vi "ByLuck.vi"(11 "InOrder":string[](array[string])) -> (3 "ByLuck":string)   [LabVIEW 2014]
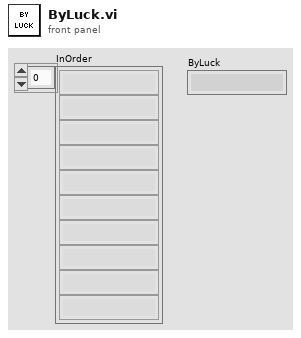
[diagram p1: front panel]
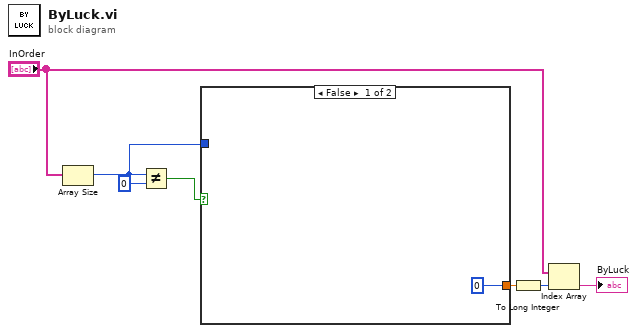
[diagram p0: block diagram]
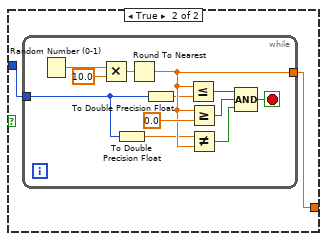
[diagram p2: hidden frame]
diagram:
  n1 = Array Size(array="InOrder") -> (size(s)=w3:i32)
  n2 = Not Equal?(x=w3, y=0) -> (x != y?=w4:bool)
  n3 = case shown="False" w4 {
    tunnel: [0 w10] -> w7
    tunnel: w3 -> [_ w9]
    frame False {
    }
    frame True {
      n4 = while {
        tunnel: w9 -> [w16]
        tunnel: [w15] -> w10
        stop <- w13 stop-if-true
        n5 = Random Number (0-1)() -> (number: 0 to 1=w22:dbl)
        n6 = Multiply(x=w22, y=10.0) -> (x*y=w20:dbl)
        n7 = To Double Precision Float(number=w16) -> (double precision float=w11:dbl)
        n8 = Round To Nearest(number=w20) -> (nearest integer value=w15:dbl)
        n9 = To Double Precision Float(number=w16) -> (double precision float=w12:dbl)
        n10 = Less Or Equal?(x=w15, y=w12) -> (x <= y?=w18:bool)
        n11 = Greater Or Equal?(x=w15, y=0.0 ("lower limit")) -> (x >= y?=w17:bool)
        n12 = Not Equal?(x=w11, y=w15) -> (x != y?=w14:bool)
        n13 = Compound Arithmetic op=AND(w18, w17, w14) -> (w13:bool)
      }
    }
  }
  n14 = To Long Integer(number=w7) -> (32bit integer=w6:i32)
  n15 = Index Array(array="InOrder", index=w6) -> (element=→"ByLuck":string)
